vi "RT_VS50_Dynamics_DLR_v3.vi"(0 "dt [s]":dbl, 1 "i":i32, 2 "Data":dbl[][](array[numeric]), 3 "V(i) [m/s]":dbl[](array[numeric]), 4 "latd(i) [rad]":dbl, 5 "lon(i) [rad]":dbl, 6 "alt(i)[m]":dbl, 7 "W_b(i) [rad/s]":dbl[](array[numeric]), 9 "W(i) [rad/s]":dbl[](array[numeric]), 11 "q(i)":dbl[](array[numeric])) -> (17 "q(i+1) 2":dbl[](array[numeric]), 18 "P(i) [m]":dbl[](array[numeric]), 19 "W(i+1) [rad/s]":dbl[](array[numeric]), 20 "Euler Angles (º)":dbl[](array[numeric]), 21 "L_C":dbl, 23 "V(i+1) [m/s]":dbl[](array[numeric]), 24 "latd(i+1) [rad]":dbl, 25 "lon(i+1)[rad]":dbl, 26 "alt(i+1) [m]":dbl, 27 "W_b(i+1) [rad/s]":dbl[](array[numeric]))   [LabVIEW 2017]
uses:
  <vilib>/Analysis/baseanly.llb/Real A x B.vi
  <vilib>/Analysis/Matrix/Numeric/Conversions/Array To Matrix - RA2.vi
  <vilib>/Analysis/Matrix/Numeric/Conversions/Array To Matrix - RA.vi
  <vilib>/Analysis/Matrix/Numeric/Conversions/Matrix To Array - RM.vi
  <vilib>/Analysis/Matrix/NI_Matrix.lvlib
  <vilib>/Analysis/NI_AALBase.lvlib
panel:
  out "M_beta":dbl
  out "M_alpha":dbl
  out "Sref [m^2]":dbl
  out "MAd [Nm]":dbl[](array[numeric])
  out "MA_f [Nm]":dbl[](array[numeric])
  in  "TVA_b":dbl[](array[numeric])
  out "MFE_b [Nm]":dbl[](array[numeric])
  out "W_b(i) [º/s]":dbl[](array[numeric])
  out "W(i) [rad/s]":dbl[](array[numeric])
  out "V(i) [m/s]":dbl[](array[numeric])
  out "ang_acc [rad/s^2]":dbl[](array[numeric])
  out "acc [m/s^2]":dbl[](array[numeric])
  out "MFA [Nm]":dbl[](array[numeric])
  out "MFE [Nm]":dbl[](array[numeric])
  out "Mco [Nm]":dbl[](array[numeric])
  out "Fco [N]":dbl[](array[numeric])
  out "FA [N]":dbl[](array[numeric])
  out "FG_b [N]":dbl[](array[numeric])
  out "FG [N]":dbl[](array[numeric])
  out "FE [N]":dbl[](array[numeric])
  out "FE_b [N]":dbl[](array[numeric])
  out "AoA_yaw [rad]":dbl
  out "AoA_pitch [rad]":dbl
  out "Patm [Pa]":dbl
  out "Pdin [Pa]":dbl
  out "Nzl_S [m^2]":dbl
  # "Forces"
  # "Time"
  # "Moments"
  # "Outputs"
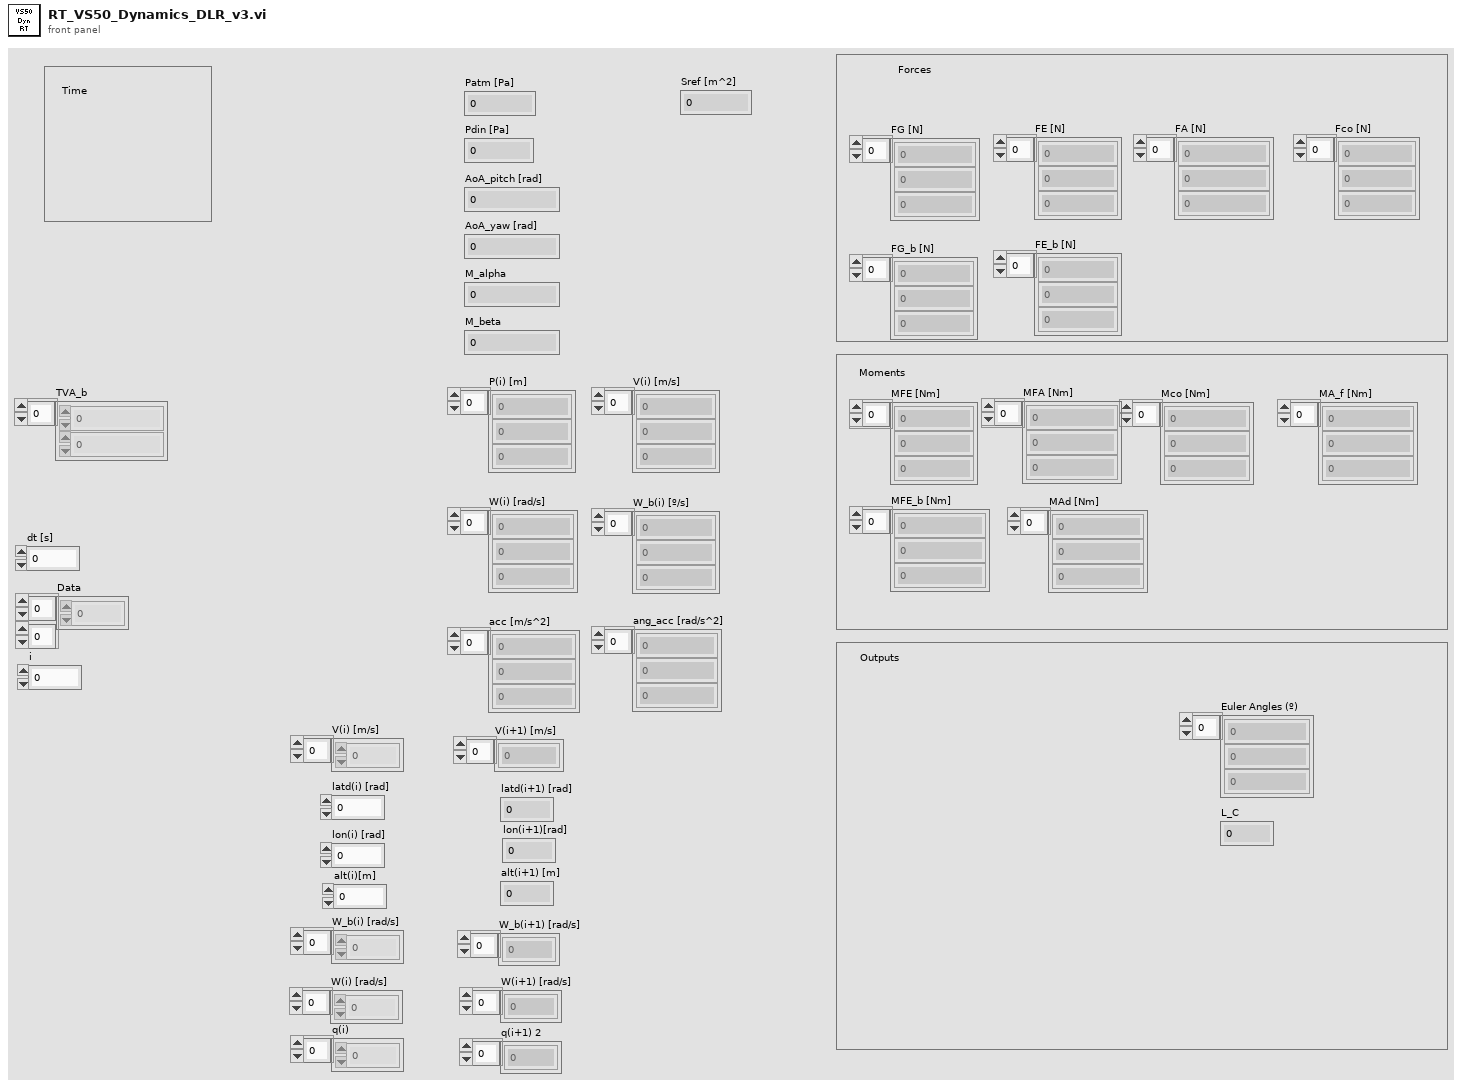
[diagram p1: front panel]
types:
  T1 = typedef "NI_Matrix.lvlib/RealMatrix.ctl" = dbl[][]
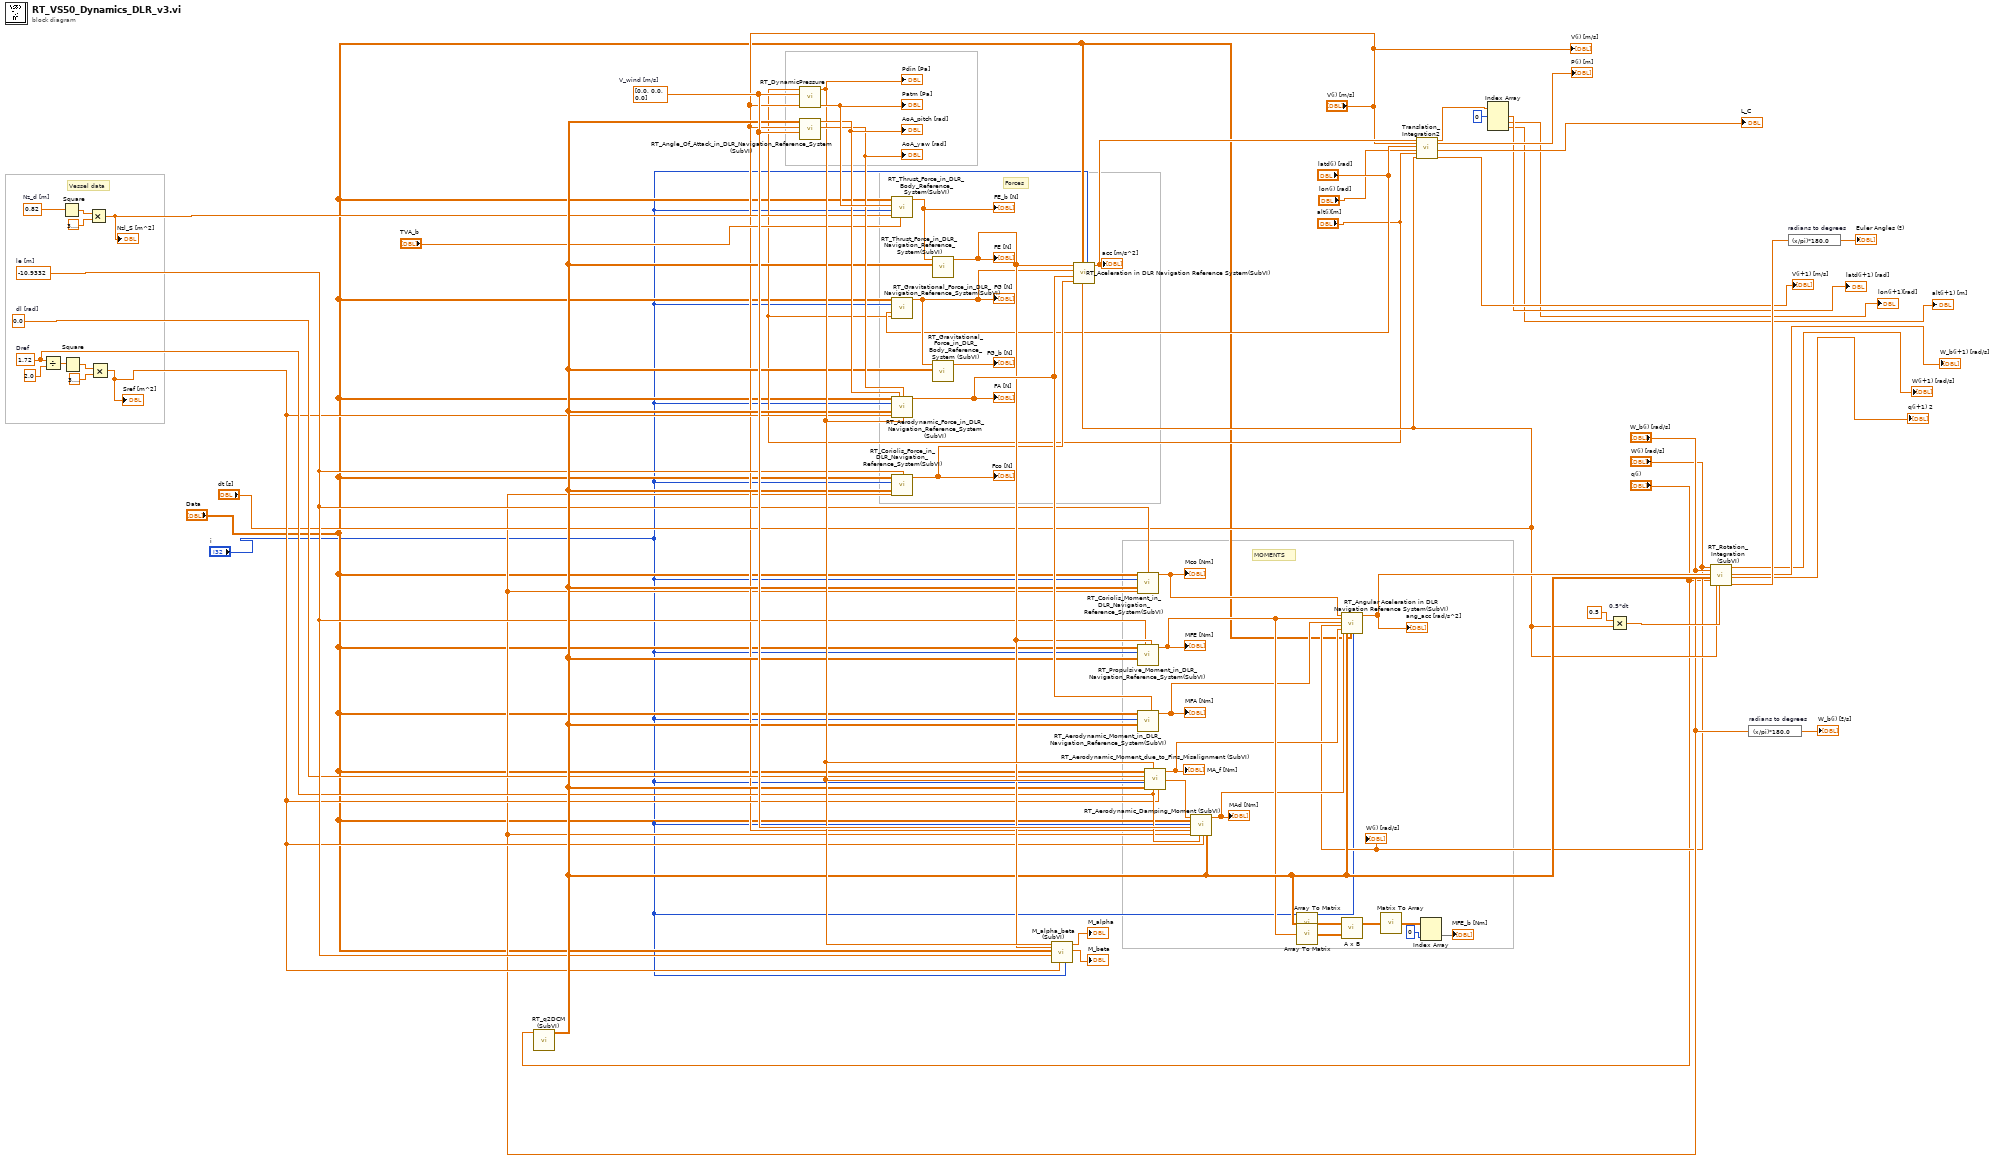
[diagram p0: block diagram]
diagram:
  w38 = 1.72  # Dref
  w39 = 0.0  # dl [rad]
  w44 = 0.82  # Nz_d [m]
  w40 = -10.9332  # le [m]
  w62 = dbl[] [0.0, 0.0, 0.0]  # V_wind [m/s]
  # "Forces"
  # "MOMENTS"
  # "Vessel data"
  n1 = Divide(x=w38, y=2.0) -> (x/y=w48:dbl)
  n2 = Square(x=w44) -> (x^2=w42:dbl)
  n3 = Square(x=w48) -> (x^2=w47:dbl)
  n4 = Multiply(x=w42, y=3.141592653589793) -> (x*y=w41:dbl)
  "Nzl_S [m^2]" <- w41
  n5 = Multiply(x=w47, y=3.141592653589793) -> (x*y=w37:dbl)
  "Sref [m^2]" <- w37
  n6 = call "RT_q2DCM (SubVI).vi"("Quaternion"="q(i)") -> ("DCM"=w49:dbl[][])  [unwired: 10 in]
  n7 = call "RT_DynamicPressure.vi"("V (m/s)"="V(i) [m/s]", "V_wind (m/s)"=w62, "h (m)"="alt(i)[m]") -> ("Patm (Pa)"=w66:dbl, "Pdin"=w61:dbl)  [unwired: 7 in]
  "Pdin [Pa]" <- w61
  "Patm [Pa]" <- w66
  n8 = call "RT_Angle_Of_Attack_in_DLR_Navigation_Reference_System (SubVI).vi"("V_wind (m/s)"=w62, "V (m/s)"="V(i) [m/s]", "DCM"=w49) -> ("AoA_yaw (rad)"=w64:dbl, "AoA_pitch (rad)"=w65:dbl)  [unwired: 7 in]
  "AoA_pitch [rad]" <- w65
  "AoA_yaw [rad]" <- w64
  n9 = call "RT_Thrust_Force_in_DLR_Body_Reference_System(SubVI).vi"("TVA_b(i)"="TVA_b", "Nzl_S"=w41, "i"="i", "Patm (Pa)"=w66, "Data"="Data") -> ("FE_b"=w10:dbl[])  [unwired: 6 in]
  "FE_b [N]" <- w10
  n10 = call "RT_Gravitational_Force_in_DLR_Navigation_Reference_System(SubVI).vi"("Data"="Data", "i"="i", "latd (rad)"="latd(i) [rad]", "alt (m)"="alt(i)[m]") -> ("FG_d"=w11:dbl[])  [unwired: 10 in, 1 out]
  "FG [N]" <- w11
  n11 = call "RT_Aerodynamic_Force_in_DLR_Navigation_Reference_System (SubVI).vi"("Data"="Data", "AoA_pitch (rad)"=w65, "AoA_yaw (rad)"=w64, "i"="i", "DCM"=w49, "Sref [m^2]"=w37, "Pdin"=w61) -> ("FA"=w60:dbl[])  [unwired: 8 in]
  "FA [N]" <- w60
  n12 = call "RT_Coriolis_Force_in_DLR_Navigation_Reference_System(SubVI).vi"("Data"="Data", "le (m) in"=w40, "i"="i", "DCM"=w49, "W_b (rad/s)"="W_b(i) [rad/s]") -> ("Fco (N)"=w12:dbl[])  [unwired: 10 in]
  "Fco [N]" <- w12
  n13 = call "RT_Thrust_Force_in_DLR_Navigation_Reference_System(SubVI).vi"("DCM"=w49, "FE_b"=w10) -> ("FE"=w59:dbl[])  [unwired: 8 in]
  "FE [N]" <- w59
  n14 = call "RT_Gravitational_Force_in_DLR_Body_Reference_System (SubVI).vi"("DCM"=w49, "FG_d"=w11) -> ("FG_b"=→"FG_b [N]":dbl[])  [unwired: 9 in]
  n15 = call "M_alpha_beta (SubVI).vi"("i"="i", "Sref"=w37, "FE [N]"=w59, "le [m]"=w40, "Data"="Data", "Pdin [Pa]"=w61) -> ("M_beta"=→"M_beta":dbl, "M_alpha"=→"M_alpha":dbl)  [unwired: 4 in]
  n16 = call "RT_Aceleration in DLR Navigation Reference System(SubVI).vi"("i"="i", "dt(s)"="dt [s]", "Data"="Data", "Fco (N)"=w12, "FA"=w60, "FG"=w11, "FE"=w59) -> ("acc"=w56:dbl[])  [unwired: 4 in]
  "acc [m/s^2]" <- w56
  n17 = call "RT_Coriolis_Moment_in_DLR_Navigation_Reference_System(SubVI).vi"("Data"="Data", "le (m) in"=w40, "i"="i", "DCM"=w49, "W_b (rad/s) in"="W_b(i) [rad/s]") -> ("Mco (Nm)"=w18:dbl[])  [unwired: 10 in]
  "Mco [Nm]" <- w18
  n18 = call "RT_Propulsive_Moment_in_DLR_Navigation_Reference_System(SubVI).vi"("FE"=w59, "le (m) in"=w40, "DCM"=w49, "i"="i", "Data"="Data") -> ("MFE (Nm)"=w17:dbl[])  [unwired: 6 in]
  "MFE [Nm]" <- w17
  n19 = call "RT_Aerodynamic_Moment_in_DLR_Navigation_Reference_System(SubVI).vi"("FA"=w60, "DCM"=w49, "i"="i", "Data"="Data") -> ("MFA (Nm)"=w16:dbl[])  [unwired: 7 in]
  "MFA [Nm]" <- w16
  n20 = call "RT_Aerodynamic_Moment_due_to_Fins_Misalignment (SubVI).vi"("Sref [m^2]"=w37, "Dref"=w38, "Pdin [Pa]"=w61, "DCM"=w49, "i"="i", "dl [rad] in"=w39, "Data"="Data") -> ("MA_f"=w15:dbl[])  [unwired: 4 in]
  "MA_f [Nm]" <- w15
  n21 = call "RT_Aerodynamic_Damping_Moment (SubVI).vi"("Pdin [Pa]"=w61, "Data"="Data", "i"="i", "V_wind [m/s]"=w62, "V(i) [m/s]"="V(i) [m/s]", "W_b(i) [º/s]"="W_b(i) [rad/s]", "Dref"=w38, "Sref [m^2]"=w37, "DCM"=w49) -> ("MAd"=w14:dbl[])  [unwired: 10 in]
  "MAd [Nm]" <- w14
  n22 = call-poly <vilib>:"Array To Matrix.vi"("Real 2D Array"=w49) -> ("Real Matrix"=w19:T1)
  n23 = call-poly <vilib>:"Array To Matrix.vi"("Real 1D Array"=w17) -> ("Real Matrix (Column Vector)"=w24:T1)
  n24 = call "RT_Angular Aceleration in DLR Navigation Reference System(SubVI).vi"("Mco (Nm)"=w18, "MFE (Nm)"=w17, "MFA (Nm)"=w16, "W (rad/s)"="W(i) [rad/s]", "MA_f [Nm]"=w15, "MAd [Nm]"=w14, "DCM"=w49, "Data"="Data", "i"="i") -> ("ang_acc"=w52:dbl[])  [unwired: 10 in]
  "ang_acc [rad/s^2]" <- w52
  n25 = call-poly <vilib>:"A x B.vi"("B"=w24, "A"=w19) -> ("A x B"=w22:T1)  [unwired: 1 out]
  n26 = call-poly <vilib>:"Matrix To Array.vi"("Real Matrix"=w22) -> ("Real 2D Array"=w23:dbl[][])
  n27 = call "Translation_Integration2.vi"("acc"=w56, "V(i) in"="V(i) [m/s]", "latd(i)"="latd(i) [rad]", "lon(i) [rad]"="lon(i) [rad]", "alt(i) [m]"="alt(i)[m]", "dt [s]"="dt [s]") -> ("position"=w53:dbl[], "position ECEF (i)"=→"P(i) [m]":dbl[], "L_C"=→"L_C":dbl, "Velocity"=→"V(i+1) [m/s]":dbl[])  [unwired: 10 in]
  n28 = Index Array(array=w23, index (col)=0 ("index (row)")) -> (element=→"MFE_b [Nm]":dbl[])  [unwired: 1 in]
  n29 = Index Array(array=w53, index #1=0 ("index")) -> (element #1=→"latd(i+1) [rad]":dbl, element #2=→"lon(i+1)[rad]":dbl, element #3=→"alt(i+1) [m]":dbl)  [unwired: 2 in]
  n30 = Multiply "0.5*dt"(x=0.5, y="dt [s]") -> (x*y=w51:dbl)
  n31 = call "RT_Rotation_Integration (SubVI).vi"("W(i) [rad/s] in"="W(i) [rad/s]", "W_b(i) [rad/s]"="W_b(i) [rad/s]", "ang_acc [rad/s^2]"=w52, "D_NB"=w49, "q(i) in"="q(i)", "dt"="dt [s]", "dt*0.5"=w51) -> ("W(i+1)"=→"W(i+1) [rad/s]":dbl[], "W_b(i+1) [rad/s]"=→"W_b(i+1) [rad/s]":dbl[], "q(i+1)"=→"q(i+1) 2":dbl[], "angles (i+1) [rad]"=w35:dbl[])  [unwired: 9 in]
  n32 = expression code="(x/pi)*180.0" "radians to degrees"("W_b(i) [rad/s]") -> (→"W_b(i) [º/s]":dbl[])
  n33 = expression code="(x/pi)*180.0" "radians to degrees"(w35) -> (→"Euler Angles (º)":dbl[])
  "V(i) [m/s]" <- "V(i) [m/s]"
  "W(i) [rad/s]" <- "W(i) [rad/s]"
